vi "VMUI_Viewer.vi"(6 "SetList VariableManager Ref in":refnum<vi>, 10 "SubPanelRef":refnum<vi>, 11 "VariableManagerRef in":refnum<vi>) -> (3 "VariableManagerRef out":refnum<vi>)   [LabVIEW 2013]
doc: "The read-only version of main user interface for VariableManager. The VariableManager should have UpdateEvent created before using this interface. See VMUIStart.vi for example."
uses:
  VariableManager/VariableManager.lvclass
  VMUI.lvclass
  <vilib>/Utility/miscctls.llb/LVRowAndColumnUnsignedTypeDef.ctl
  <vilib>/Utility/miscctls.llb/LVRowAndColumnTypeDef.ctl
  API/VariableManagerAPI.lvlib
panel:
  out "SetList Variables\nrefnum invalid?":bool
  in  "VMUI":refnum<class "VMUI.lvclass">
  in  "Variable Group":u16(ring) items=["All"]
  in  "Variables":string[][](table)
  in  "EvaluateSquenceValues":bool
  in  "Sequence Indices":string[][](table)
  in  "Sequence Values":string[][](table) caption="Sequence Status"
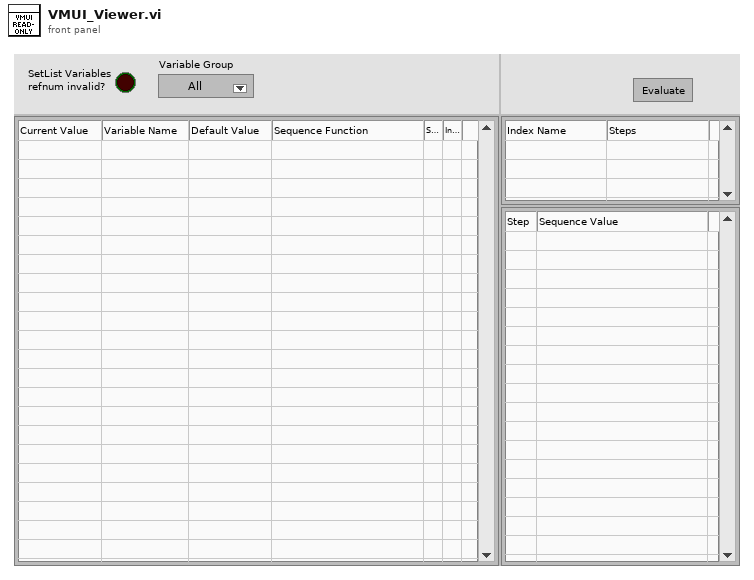
[diagram p1: front panel]
types:
  T1 = typedef "LVRowAndColumnUnsignedTypeDef.ctl" = cluster{"Row":u32, "Column":u32}
  T2 = typedef "LVRowAndColumnTypeDef.ctl" = cluster{"Row":i32, "Column":i32}
  T3 = typedef "LVPoint32TypeDef.ctl" = cluster{"Horizontal":i32, "Vertical":i32}
  T4 = typedef "LVRectTypeDef.ctl" = cluster{"Left":i16, "Top":i16, "Right":i16, "Bottom":i16}
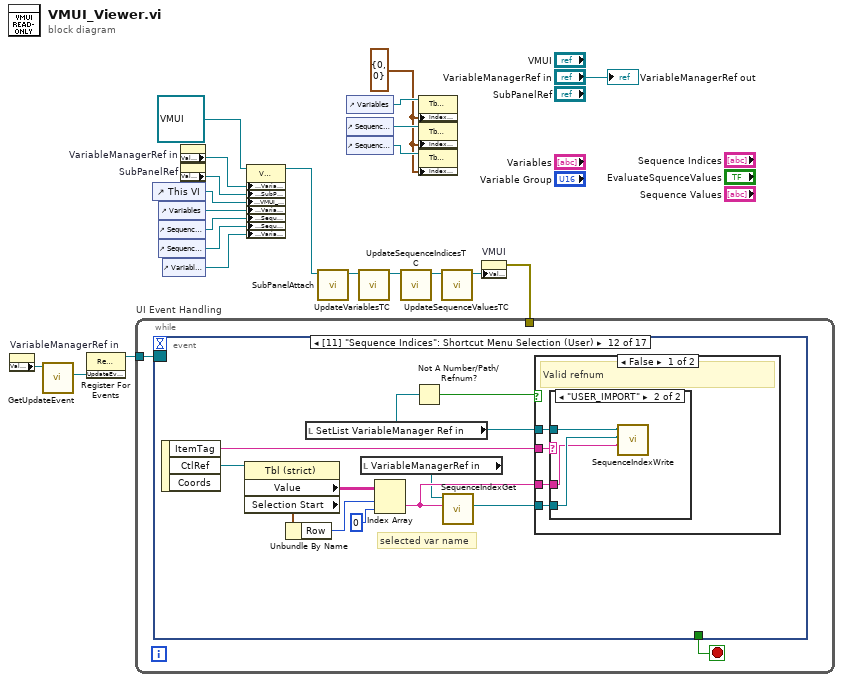
[diagram p0: block diagram]
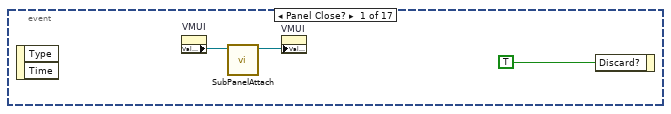
[diagram p2: hidden frame]
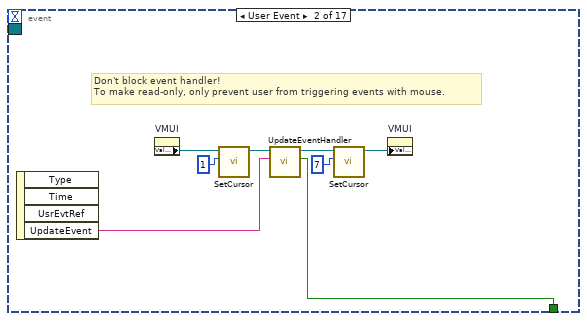
[diagram p3: hidden frame]
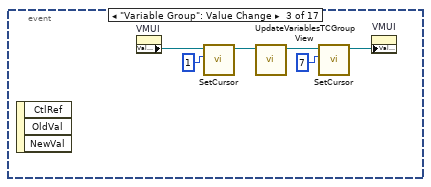
[diagram p4: hidden frame]
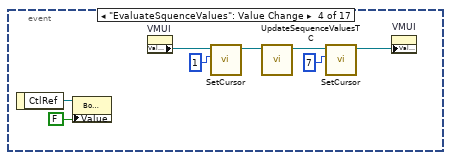
[diagram p5: hidden frame]
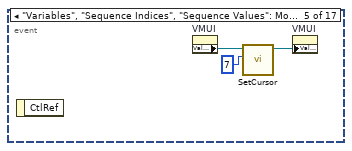
[diagram p6: hidden frame]
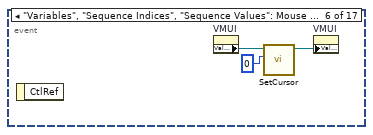
[diagram p7: hidden frame]
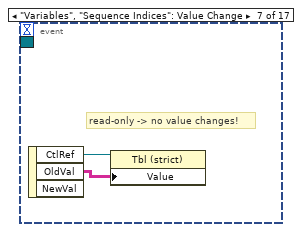
[diagram p8: hidden frame]
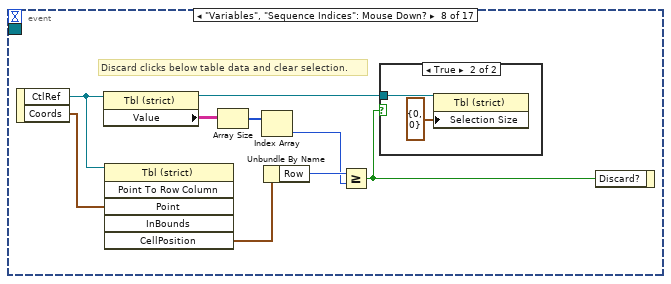
[diagram p9: hidden frame]
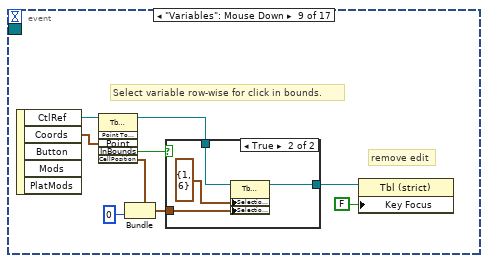
[diagram p11: hidden frame]
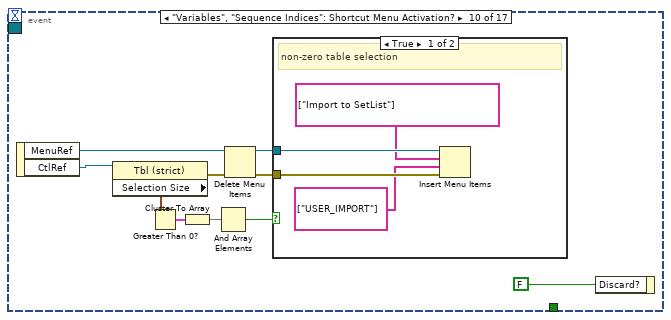
[diagram p13: hidden frame]
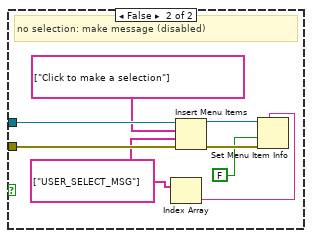
[diagram p14: hidden frame]
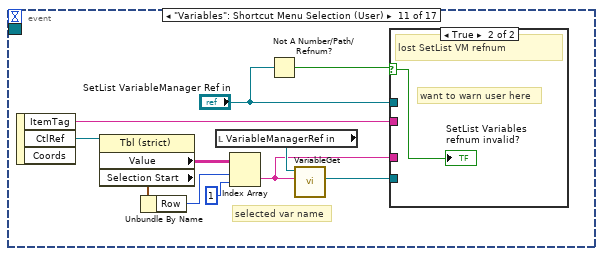
[diagram p15: hidden frame]
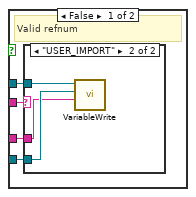
[diagram p16: hidden frame]
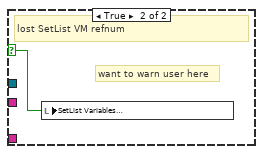
[diagram p19: hidden frame]
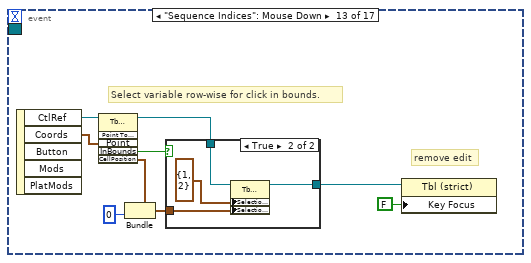
[diagram p20: hidden frame]
diagram:
  w2 = T1 {"Row"=0, "Column"=0} ("Index Values")
  n1 = property on="VariableManagerRef in" class="LVObjRef (strict)"() -> ("Value"=w13:refnum<vi>)  [unwired: 2 in, 2 out]
  n2 = call "GetUpdateEvent.vi"("VariableManagerRef in"=w13) -> ("UpdateEvent"=w12:refnum<user-event>)  [unwired: 8 in, 2 out]
  n3 = register-events(w12) -> (reference out=w11:refnum<event-registration>)  [unwired: 2 in, 1 out]
  n4 = control-ref of="This VI"() -> (w18:refnum<vi>)
  n5 = control-ref of="Variables"() -> (w17:refnum<vi>)
  n6 = control-ref of="Sequence Indices"() -> (w16:refnum<vi>)
  n7 = control-ref of="Sequence Values"() -> (w15:refnum<vi>)
  n8 = control-ref of="Variable Group"() -> (w14:refnum<vi>)
  n9 = property on="VariableManagerRef in" class="LVObjRef (strict)"() -> ("Value"=w20:refnum<vi>)  [unwired: 2 in, 2 out]
  n10 = property on="SubPanelRef" class="LVObjRef (strict)"() -> ("Value"=w19:refnum<vi>)  [unwired: 2 in, 2 out]
  n11 = property class="VMUI.lvclass"(reference=refnum<class "VMUI.lvclass"> refnum ("VMUI.lvclass"), "Accessors:VariableManagerRef"=w20, "Accessors:SubPanelRef"=w19, "Accessors:VMUI_VI_Ref"=w18, "Accessors:VariablesTCRef"=w17, "Accessors:SequenceIndicesTCRef"=w16, "Accessors:SequenceValuesTCRef"=w15, "Accessors:VariableGroupRingRef"=w14) -> (reference out=w10:refnum<class "VMUI.lvclass">)  [unwired: 1 in, 1 out]
  n12 = call-dynamic "SubPanelAttach.vi"("VMUI in"=w10) -> ("VMUI out"=w9:refnum<class "VMUI.lvclass">)  [unwired: 9 in, 1 out]
  n13 = control-ref of="Variables"() -> (w5:refnum<vi>)
  n14 = control-ref of="Sequence Indices"() -> (w3:refnum<vi>)
  n15 = control-ref of="Sequence Values"() -> (w4:refnum<vi>)
  n16 = call-dynamic "UpdateVariablesTC.vi"("VMUI in"=w9) -> ("VMUI out"=w8:refnum<class "VMUI.lvclass">)  [unwired: 9 in, 1 out]
  n17 = call-dynamic "UpdateSequenceIndicesTC.vi"("VMUI in"=w8) -> ("VMUI out"=w7:refnum<class "VMUI.lvclass">)  [unwired: 9 in, 1 out]
  n18 = property class="Tbl (strict)"(reference=w5, "Index Values"=w2) -> ()  [unwired: 1 in, 2 out]
  n19 = property class="Tbl (strict)"(reference=w3, "Index Values"=w2) -> ()  [unwired: 1 in, 2 out]
  n20 = property class="Tbl (strict)"(reference=w4, "Index Values"=w2) -> ()  [unwired: 1 in, 2 out]
  n21 = call-dynamic "UpdateSequenceValuesTC.vi"("VMUI in"=w7) -> ("VMUI out"=w6:refnum<class "VMUI.lvclass">)  [unwired: 9 in, 1 out]
  n22 = property on="VMUI" class="LVClassControl (strict)"("Value"=w6) -> (error out=w1:errorcluster)  [unwired: 2 in, 1 out]
  n23 = while "UI Event Handling" {
    tunnel: w11 -> [w24]
    tunnel: w1 -> [_]
    stop <- w23 stop-if-true
    n24 = event shown="[11] \"Sequence Indices\": Shortcut Menu Selection (User)" {
      selector: w24 -> [_ _ _ _ _ _ _ _ _ _ _ _ _ _ _ _ _]
      dyn-events: _ -> [_ _ _ _ _ _ _ _ _ _ _ _ _ _ _ _ _]
      timeout: _ -> [_ _ _ _ _ _ _ _ _ _ _ _ _ _ _ _ _]
      tunnel: [_ w35 _ _ _ _ _ _ _ _ _ _ _ _ _ _ _] -> w23
      event Panel Close? {
        n25 = event-data() -> ()  [unwired: 1 in, 2 out]
        n26 = property on="VMUI" class="LVClassControl (strict)"() -> ("Value"=w26:refnum<class "VMUI.lvclass">)  [unwired: 2 in, 2 out]
        n27 = call-dynamic "SubPanelAttach.vi"("VMUI in"=w26) -> ("VMUI out"=w25:refnum<class "VMUI.lvclass">)  [unwired: 9 in, 1 out]
        n28 = property on="VMUI" class="LVClassControl (strict)"("Value"=w25) -> ()  [unwired: 2 in, 2 out]
        n29 = event-data("Discard?"=TRUE) -> ()  [unwired: 1 in, 1 out]
      }
      event User Event {
        # "Don't block event handler!\nTo make read-only, only prevent user from triggering events with mouse."
        n30 = event-data() -> ("UpdateEvent"=w34:string)  [unwired: 1 in, 3 out]
        n31 = property on="VMUI" class="LVClassControl (strict)"() -> ("Value"=w31:refnum<class "VMUI.lvclass">)  [unwired: 2 in, 2 out]
        n32 = call-dynamic "SetCursor.vi"("icon"=u16 1, "VMUI in"=w31) -> ("VMUI out"=w30:refnum<class "VMUI.lvclass">)  [unwired: 8 in, 1 out]
        n33 = call-dynamic "UpdateEventHandler.vi"("UpdateEvent"=w34, "VMUI in"=w30) -> ("Stop"=w35:bool, "VMUI out"=w29:refnum<class "VMUI.lvclass">)  [unwired: 7 in, 1 out]
        n34 = call-dynamic "SetCursor.vi"("icon"=u16 7, "VMUI in"=w29) -> ("VMUI out"=w28:refnum<class "VMUI.lvclass">)  [unwired: 8 in, 1 out]
        n35 = property on="VMUI" class="LVClassControl (strict)"("Value"=w28) -> ()  [unwired: 2 in, 2 out]
      }
      event "Variable Group": Value Change {
        n36 = event-data() -> ()  [unwired: 1 in, 3 out]
        n37 = property on="VMUI" class="LVClassControl (strict)"() -> ("Value"=w39:refnum<class "VMUI.lvclass">)  [unwired: 2 in, 2 out]
        n38 = call-dynamic "SetCursor.vi"("icon"=u16 1, "VMUI in"=w39) -> ("VMUI out"=w38:refnum<class "VMUI.lvclass">)  [unwired: 8 in, 1 out]
        n39 = call-dynamic "UpdateVariablesTCGroupView.vi"("VMUI in"=w38) -> ("VMUI out"=w37:refnum<class "VMUI.lvclass">)  [unwired: 9 in, 1 out]
        n40 = call-dynamic "SetCursor.vi"("icon"=u16 7, "VMUI in"=w37) -> ("VMUI out"=w36:refnum<class "VMUI.lvclass">)  [unwired: 8 in, 1 out]
        n41 = property on="VMUI" class="LVClassControl (strict)"("Value"=w36) -> ()  [unwired: 2 in, 2 out]
      }
      event "EvaluateSquenceValues": Value Change {
        n42 = event-data() -> ("CtlRef"=w49:refnum<vi>)  [unwired: 1 in]
        n43 = property class="Bool (strict)"(reference=w49, "Value"=FALSE) -> ()  [unwired: 1 in, 2 out]
        n44 = property on="VMUI" class="LVClassControl (strict)"() -> ("Value"=w45:refnum<class "VMUI.lvclass">)  [unwired: 2 in, 2 out]
        n45 = call-dynamic "SetCursor.vi"("icon"=u16 1, "VMUI in"=w45) -> ("VMUI out"=w44:refnum<class "VMUI.lvclass">)  [unwired: 8 in, 1 out]
        n46 = call-dynamic "UpdateSequenceValuesTC.vi"("VMUI in"=w44) -> ("VMUI out"=w43:refnum<class "VMUI.lvclass">)  [unwired: 9 in, 1 out]
        n47 = call-dynamic "SetCursor.vi"("icon"=u16 7, "VMUI in"=w43) -> ("VMUI out"=w42:refnum<class "VMUI.lvclass">)  [unwired: 8 in, 1 out]
        n48 = property on="VMUI" class="LVClassControl (strict)"("Value"=w42) -> ()  [unwired: 2 in, 2 out]
      }
      event "Variables", "Sequence Indices", "Sequence Values": Mouse Enter {
        n49 = event-data() -> ()  [unwired: 1 in, 1 out]
        n50 = property on="VMUI" class="LVClassControl (strict)"() -> ("Value"=w52:refnum<class "VMUI.lvclass">)  [unwired: 2 in, 2 out]
        n51 = call-dynamic "SetCursor.vi"("icon"=u16 7, "VMUI in"=w52) -> ("VMUI out"=w51:refnum<class "VMUI.lvclass">)  [unwired: 8 in, 1 out]
        n52 = property on="VMUI" class="LVClassControl (strict)"("Value"=w51) -> ()  [unwired: 2 in, 2 out]
      }
      event "Variables", "Sequence Indices", "Sequence Values": Mouse Leave {
        n53 = event-data() -> ()  [unwired: 1 in, 1 out]
        n54 = property on="VMUI" class="LVClassControl (strict)"() -> ("Value"=w55:refnum<class "VMUI.lvclass">)  [unwired: 2 in, 2 out]
        n55 = call-dynamic "SetCursor.vi"("icon"=u16 0, "VMUI in"=w55) -> ("VMUI out"=w54:refnum<class "VMUI.lvclass">)  [unwired: 8 in, 1 out]
        n56 = property on="VMUI" class="LVClassControl (strict)"("Value"=w54) -> ()  [unwired: 2 in, 2 out]
      }
      event "Variables", "Sequence Indices": Value Change {
        # "read-only -> no value changes!"
        n57 = event-data() -> ("CtlRef"=w57:refnum<vi>, "OldVal"=w56:string[][])  [unwired: 1 in, 1 out]
        n58 = property class="Tbl (strict)"(reference=w57, "Value"=w56) -> ()  [unwired: 1 in, 2 out]
      }
      event "Variables", "Sequence Indices": Mouse Down? {
        # "Discard clicks below table data and clear selection."
        n59 = event-data() -> ("CtlRef"=w64:refnum<vi>, "Coords"=w63:T3)  [unwired: 1 in]
        n60 = property class="Tbl (strict)"(reference=w64) -> (reference out=w59:refnum<vi>, "Value"=w66:string[][])  [unwired: 1 in, 1 out]
        n61 = invoke class="Tbl (strict)" method="Point To Row Column"(reference=w64, "Point"=w63) -> ("CellPosition"=w62:T2)  [unwired: 4 in, 5 out]
        n62 = Array Size(array=w66) -> (size(s)=w65:i32[])
        n63 = Index Array(array=w65) -> (element=w60:i32)  [unwired: 1 in]
        n64 = Unbundle By Name(w62) -> ("Row"=w61:i32)
        n65 = Greater Or Equal?(x=w61, y=w60) -> (x >= y?=w58:bool)
        n66 = case shown="True" w58 {
          tunnel: w59 -> [_ w68]
          frame False {
          }
          frame True {
            n67 = property class="Tbl (strict)"(reference=w68, "Selection Size"=T2 {"Row"=0, "Column"=0}) -> ()  [unwired: 1 in, 2 out]
          }
        }
        n68 = event-data("Discard?"=w58) -> ()  [unwired: 1 in, 1 out]
      }
      event "Variables": Mouse Down {
        # "remove edit"
        # "Select variable row-wise for click in bounds."
        n69 = event-data() -> ("CtlRef"=w77:refnum<vi>, "Coords"=w76:T3)  [unwired: 1 in, 3 out]
        n70 = invoke class="Tbl (strict)" method="Point To Row Column"(reference=w77, "Point"=w76) -> (reference out=w74:refnum<vi>, "InBounds"=w75:bool, "CellPosition"=w72:T2)  [unwired: 4 in, 3 out]
        n71 = Bundle(cluster=w72, "Column"=0) -> (w71:T2)  [unwired: 1 in]
        n72 = case shown="True" w75 {
          tunnel: w71 -> [_ w81]
          tunnel: w74 -> [w78 w80]
          tunnel: [w78 w79] -> w70
          frame False {
          }
          frame True {
            n73 = property class="Tbl (strict)"(reference=w80, "Selection Size"=T2 {"Row"=1, "Column"=6}, "Selection Start"=w81) -> (reference out=w79:refnum<vi>)  [unwired: 1 in, 1 out]
          }
        }
        n74 = property class="Tbl (strict)"(reference=w70, "Key Focus"=FALSE) -> ()  [unwired: 1 in, 2 out]
      }
      event "Variables", "Sequence Indices": Shortcut Menu Activation? {
        n75 = event-data() -> ("MenuRef"=w85:refnum<k9>, "CtlRef"=w84:refnum<vi>)  [unwired: 1 in]
        n76 = property class="Tbl (strict)"(reference=w84) -> (error out=w89:errorcluster, "Selection Size"=w92:T2)  [unwired: 1 in, 1 out]
        n77 = Greater Than 0?(x=w92) -> (x > 0?=w91:cluster{"Row":bool, "Column":bool})
        n78 = Cluster To Array(cluster=w91) -> (array=w90:bool[])
        n79 = And Array Elements(Boolean array=w90) -> (logical AND=w86:bool)
        n80 = Delete Menu Items(6:w89, 9:w85) -> (0:w88:errorcluster, 3:w87:refnum<k9>)  [unwired: 2 in]
        n81 = case shown="True" w86 {
          tunnel: w88 -> [w96 w104]
          tunnel: w87 -> [w95 w103]
          frame True {
            # "non-zero table selection"
            n82 = Insert Menu Items(6:w96, 7:string[] ["USER_IMPORT"] ("item names"), 8:string[] ["Import to SetList"] ("item names"), 9:w95) -> ()  [unwired: 2 in, 3 out]
          }
          frame False {
            w99 = string[] ["USER_SELECT_MSG"] ("item names")
            # "no selection: make message (disabled)"
            n83 = Index Array(array=w99) -> (element=w98:string)  [unwired: 1 in]
            n84 = Insert Menu Items(6:w104, 7:w99, 8:string[] ["Click to make a selection"] ("item names"), 9:w103) -> (0:w102:errorcluster, 3:w97:refnum<k9>)  [unwired: 2 in, 1 out]
            n85 = Set Menu Item Info(7:w98, 8:w102, 9:FALSE ("enabled"), 11:w97) -> ()  [unwired: 3 in, 2 out]
          }
        }
        n86 = event-data("Discard?"=FALSE) -> ()  [unwired: 1 in, 1 out]
      }
      event "Variables": Shortcut Menu Selection (User) {
        # "selected var name"
        n87 = event-data() -> ("ItemTag"=w115:string, "CtlRef"=w114:refnum<vi>)  [unwired: 1 in, 1 out]
        n88 = property class="Tbl (strict)"(reference=w114) -> ("Value"=w113:string[][], "Selection Start"=w112:T2)  [unwired: 1 in, 2 out]
        n89 = Unbundle By Name(w112) -> ("Row"=w111:i32)
        n90 = local read "VariableManagerRef in"() -> (w109:refnum<vi>)
        n91 = Index Array(array=w113, index (row)=w111, index (col)=1 ("disabled index (col)")) -> (element=w107:string)
        n92 = Not A Number/Path/Refnum?(number/path/refnum="SetList VariableManager Ref in") -> (NaN/Path/Refnum?=w105:bool)
        n93 = call "VariableGet.vi"("VariableName"=w107, "VariableManagerRef in"=w109) -> ("Variable"=w108:refnum<class "Variable.lvclass">)  [unwired: 7 in, 2 out]
        n94 = case shown="True" w105 {
          selector: w105 -> [_ w123]
          tunnel: w115 -> [w119 _]
          tunnel: w108 -> [w118 _]
          tunnel: w107 -> [w117 _]
          tunnel: "SetList VariableManager Ref in" -> [w116 _]
          frame False {
            # "Valid refnum"
            n95 = case shown="\"USER_IMPORT\"" w119 {
              tunnel: w116 -> [_ w121]
              tunnel: w118 -> [_ w122]
              tunnel: w117 -> [_ w120]
              frame Default {
              }
              frame "USER_IMPORT" {
                n96 = call "VariableWrite.vi"("OriginalName"=w120, "Variable"=w122, "VariableManagerRef in"=w121) -> ()  [unwired: 7 in, 2 out]
              }
            }
          }
          frame True {
            # "want to warn user here"
            # "lost SetList VM refnum"
            "SetList Variables\nrefnum invalid?" <- w123
          }
        }
      }
      event "Sequence Indices": Shortcut Menu Selection (User) {
        # "selected var name"
        n97 = event-data() -> ("ItemTag"=w134:string, "CtlRef"=w133:refnum<vi>)  [unwired: 1 in, 1 out]
        n98 = property class="Tbl (strict)"(reference=w133) -> ("Value"=w132:string[][], "Selection Start"=w131:T2)  [unwired: 1 in, 2 out]
        n99 = Unbundle By Name(w131) -> ("Row"=w130:i32)
        n100 = local read "SetList VariableManager Ref in"() -> (w127:refnum<vi>)
        n101 = local read "VariableManagerRef in"() -> (w125:refnum<vi>)
        n102 = Index Array(array=w132, index (row)=w130, index (col)=0 ("disabled index (col)")) -> (element=w126:string)
        n103 = Not A Number/Path/Refnum?(number/path/refnum=w127) -> (NaN/Path/Refnum?=w128:bool)
        n104 = call "SequenceIndexGet.vi"("SequenceIndexName"=w126, "VariableManagerRef in"=w125) -> ("SequenceIndex"=w124:refnum<class "SequenceIndex.lvclass">)  [unwired: 7 in, 2 out]
        n105 = case shown="False" w128 {
          selector: w128 -> [_ w142]
          tunnel: w134 -> [w138 _]
          tunnel: w124 -> [w137 _]
          tunnel: w126 -> [w136 _]
          tunnel: w127 -> [w135 _]
          frame False {
            # "Valid refnum"
            n106 = case shown="\"USER_IMPORT\"" w138 {
              tunnel: w135 -> [_ w141]
              tunnel: w137 -> [_ w140]
              tunnel: w136 -> [_ w139]
              frame Default {
              }
              frame "USER_IMPORT" {
                n107 = call "SequenceIndexWrite.vi"("OriginalName"=w139, "SequenceIndex"=w140, "VariableManagerRef in"=w141) -> ()  [unwired: 7 in, 2 out]
              }
            }
          }
          frame True {
            # "want to warn user here"
            # "lost SetList VM refnum"
            n108 = local write "SetList Variables\nrefnum invalid?"(w142) -> ()
          }
        }
      }
      event "Sequence Indices": Mouse Down {
        # "remove edit"
        # "Select variable row-wise for click in bounds."
        n109 = event-data() -> ("CtlRef"=w149:refnum<vi>, "Coords"=w148:T3)  [unwired: 1 in, 3 out]
        n110 = invoke class="Tbl (strict)" method="Point To Row Column"(reference=w149, "Point"=w148) -> (reference out=w150:refnum<vi>, "InBounds"=w151:bool, "CellPosition"=w147:T2)  [unwired: 4 in, 3 out]
        n111 = Bundle(cluster=w147, "Column"=0) -> (w145:T2)  [unwired: 1 in]
        n112 = case shown="True" w151 {
          tunnel: w145 -> [_ w155]
          tunnel: w150 -> [w152 w154]
          tunnel: [w152 w153] -> w143
          frame False {
          }
          frame True {
            n113 = property class="Tbl (strict)"(reference=w154, "Selection Size"=T2 {"Row"=1, "Column"=2}, "Selection Start"=w155) -> (reference out=w153:refnum<vi>)  [unwired: 1 in, 1 out]
          }
        }
        n114 = property class="Tbl (strict)"(reference=w143, "Key Focus"=FALSE) -> ()  [unwired: 1 in, 2 out]
      }
      event "Sequence Values": Mouse Down? {
        w157 = T2 {"Row"=0, "Column"=0} ("Selection Start")
        # "only clicks allowed: left click on scroll bar."
        n115 = event-data() -> ("CtlRef"=w165:refnum<vi>, "Coords"=w164:T3, "Button"=w161:u16)  [unwired: 1 in, 2 out]
        n116 = Not Equal?(x=w161, y=u16 1) -> (x != y?=w159:bool)
        n117 = invoke class="Tbl (strict)" method="Point To Row Column"(reference=w165, "Point"=w164) -> (reference out=w163:refnum<vi>, "InBounds"=w160:bool)  [unwired: 4 in, 4 out]
        n118 = Or(x=w160, y=w159) -> (x .or. y?=w158:bool)
        n119 = property class="Tbl (strict)"(reference=w163, "Selection Size"=w157, "Selection Start"=w157) -> ()  [unwired: 1 in, 2 out]
        n120 = event-data("Discard?"=w158) -> ()  [unwired: 4 in, 1 out]
      }
      event Pane Size {
        n121 = event-data() -> ("NewBnds"=w167:T4)  [unwired: 1 in, 2 out]
        n122 = Unbundle(w167) -> ("Left"=w169:i16, "Right"=w168:i16)  [unwired: 2 out]
        n123 = Subtract(x=w168, y=w169) -> (x-y=w171:i16)
        n124 = control-ref of="Variables"() -> (w166:refnum<vi>)
        n125 = Subtract(x=w171, y=i16 64) -> (x-y=w173:i16)
        n126 = Quotient & Remainder(x=w173, y=i16 5) -> (floor(x/y)=w175:i16)  [unwired: 1 out]
        n127 = for {
          N: 6 -> [_]
          tunnel: w175 -> [w177]
          tunnel: w166 -> [w176]
          i -> [w178]
          n128 = case shown="4, 5" w178 {
            selector: w178 -> [_ w182 w189 w194]
            tunnel: w177 -> [_ w180 w186 _]
            tunnel: w176 -> [_ w179 w187 w191]
            frame Default {
            }
            frame 0..2 {
              n129 = Bundle By Name(cluster=T2 {"Row"=-2, "Column"=0} ("Active Cell:Active Cell"), "Column"=w182) -> (w181:T2)
              n130 = property class="Tbl (strict)"(reference=w179, "Active Cell"=w181, "Width"=w180) -> ()  [unwired: 1 in, 2 out]
            }
            frame 3 {
              n131 = Bundle By Name(cluster=T2 {"Row"=-2, "Column"=0} ("Active Cell:Active Cell"), "Column"=w189) -> (w188:T2)
              n132 = Multiply(x=w186, y=i16 2) -> (x*y=w185:i16)
              n133 = property class="Tbl (strict)"(reference=w187, "Active Cell"=w188, "Width"=w185) -> ()  [unwired: 1 in, 2 out]
            }
            frame 4, 5 {
              n134 = Bundle By Name(cluster=T2 {"Row"=-2, "Column"=0} ("Active Cell:Active Cell"), "Column"=w194) -> (w193:T2)
              n135 = property class="Tbl (strict)"(reference=w191, "Active Cell"=w193, "Width"=u32 17 ("Active Cell:Cell Size:Width")) -> ()  [unwired: 1 in, 2 out]
            }
          }
        }
      }
      event Pane Size {
        n136 = event-data() -> ("NewBnds"=w197:T4)  [unwired: 1 in, 2 out]
        n137 = Unbundle(w197) -> ("Left"=w199:i16, "Right"=w198:i16)  [unwired: 2 out]
        n138 = Subtract(x=w198, y=w199) -> (x-y=w201:i16)
        n139 = control-ref of="Sequence Indices"() -> (w196:refnum<vi>)
        n140 = Subtract(x=w201, y=i16 30) -> (x-y=w203:i16)
        n141 = Quotient & Remainder(x=w203, y=i16 2) -> (floor(x/y)=w205:i16)  [unwired: 1 out]
        n142 = for {
          N: 2 -> [_]
          tunnel: w205 -> [w207]
          tunnel: w196 -> [w206]
          i -> [w208]
          n143 = case shown="0, 1" w208 {
            selector: w208 -> [_ w212]
            tunnel: w207 -> [_ w209]
            tunnel: w206 -> [_ w210]
            frame Default {
            }
            frame 0, 1 {
              n144 = Bundle By Name(cluster=T2 {"Row"=-2, "Column"=0} ("Active Cell:Active Cell"), "Column"=w212) -> (w211:T2)
              n145 = property class="Tbl (strict)"(reference=w210, "Active Cell"=w211, "Width"=w209) -> ()  [unwired: 1 in, 2 out]
            }
          }
        }
      }
      event Pane Size {
        n146 = event-data() -> ("NewBnds"=w215:T4)  [unwired: 1 in, 2 out]
        n147 = Unbundle(w215) -> ("Left"=w217:i16, "Right"=w216:i16)  [unwired: 2 out]
        n148 = Subtract(x=w216, y=w217) -> (x-y=w219:i16)
        n149 = control-ref of="Sequence Values"() -> (w214:refnum<vi>)
        n150 = Subtract(x=w219, y=i16 60) -> (x-y=w221:i16)
        n151 = for {
          N: 2 -> [_]
          tunnel: w221 -> [w223]
          tunnel: w214 -> [w222]
          i -> [w224]
          n152 = case shown="0" w224 {
            selector: w224 -> [_ w228 w233]
            tunnel: w223 -> [_ _ w230]
            tunnel: w222 -> [_ w226 w231]
            frame Default {
            }
            frame 0 {
              n153 = Bundle By Name(cluster=T2 {"Row"=-2, "Column"=0} ("Active Cell:Active Cell"), "Column"=w228) -> (w227:T2)
              n154 = property class="Tbl (strict)"(reference=w226, "Active Cell"=w227, "Width"=u32 30 ("Active Cell:Cell Size:Width")) -> ()  [unwired: 1 in, 2 out]
            }
            frame 1 {
              n155 = Bundle By Name(cluster=T2 {"Row"=-2, "Column"=0} ("Active Cell:Active Cell"), "Column"=w233) -> (w232:T2)
              n156 = property class="Tbl (strict)"(reference=w231, "Active Cell"=w232, "Width"=w230) -> ()  [unwired: 1 in, 2 out]
            }
          }
        }
      }
    }
  }
  "VariableManagerRef out" <- "VariableManagerRef in"
